vi "MCCETC03_Main.vi"() -> ()   [LabVIEW 2019]
uses:
  MCCETC_Global.vi
panel:
  out "T7":dbl format="%.2f"
  out "T6":dbl format="%.2f"
  out "T5":dbl format="%.2f"
  out "T4":dbl format="%.2f"
  in  "Logging":bool=TRUE
  out "status_rec":bool caption="Logging Status"
  out "T3":dbl format="%.2f"
  out "T2":dbl format="%.2f"
  in  "Tab Control":T1(tab)
  out "T0 Chart":waveform(dbl)[](graph)
  out "T1 Chart":waveform(dbl)[](graph)
  out "T2 Chart":waveform(dbl)[](graph)
  out "T3 Chart":waveform(dbl)[](graph)
  out "status_dio":bool caption="DIO Control Status"
  in  "degC_low":dbl=5.0 caption="From"
  in  "degC_hi":dbl=45.0 caption="To"
  out "alarm_t":bool caption="Temperature Alarm"
  out "T5 Chart":waveform(dbl)[](graph)
  out "T4 Chart":waveform(dbl)[](graph)
  out "T6 Chart":waveform(dbl)[](graph)
  out "T7 Chart":waveform(dbl)[](graph)
  in  "Readout Interval":i32=5 caption="sec"
  out "T1":dbl format="%.2f"
  out "T0":dbl format="%.2f"
  out "Readout Status":bool
  out "Last Measured":timestamp format="%<%Y-%m-%d %H:%M:%S>T"
  in  "stop":bool
  # "MCC E-TC #03:  Thermocouples for Annealing & Microwave Control Systems"
  # "Annealing System"
  # "K"
  # "K"
  # "Microwave System"
  # "°C"
  # "EIO Tube"
  # "EIO Top"
  # "°C"
  # "North He Riser:"
  # "°C"
  # "IVC Top:"
  # "°C"
  # "Heat Tape: IVC:"
  # "°F"
  # "Heat Tape: Turret:"
  # "°F"
  # "Good Temperature Range (degC)"
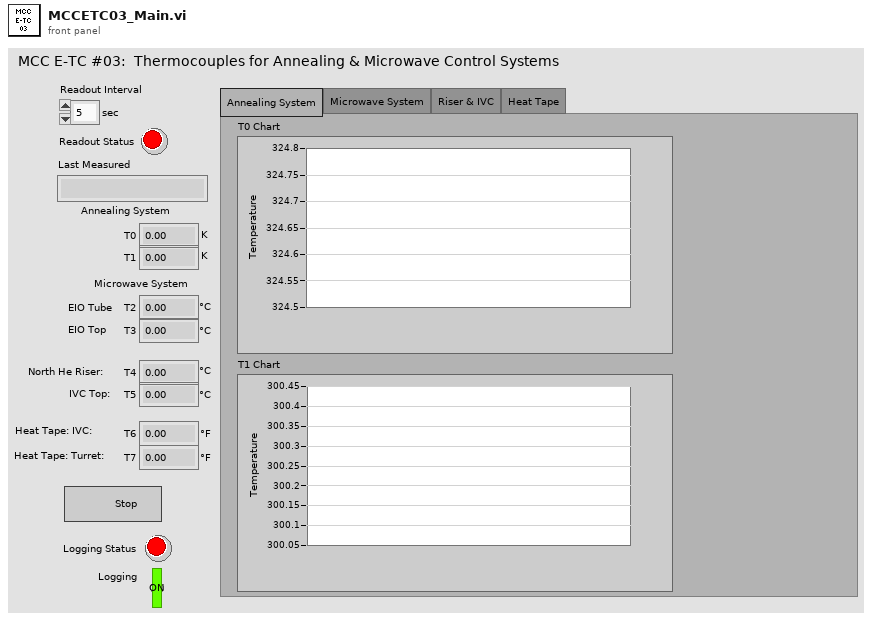
[diagram p1: front panel]
types:
  T1 = enum32{"Annealing System", "Microwave System", "Riser & IVC", "Heat Tape"}
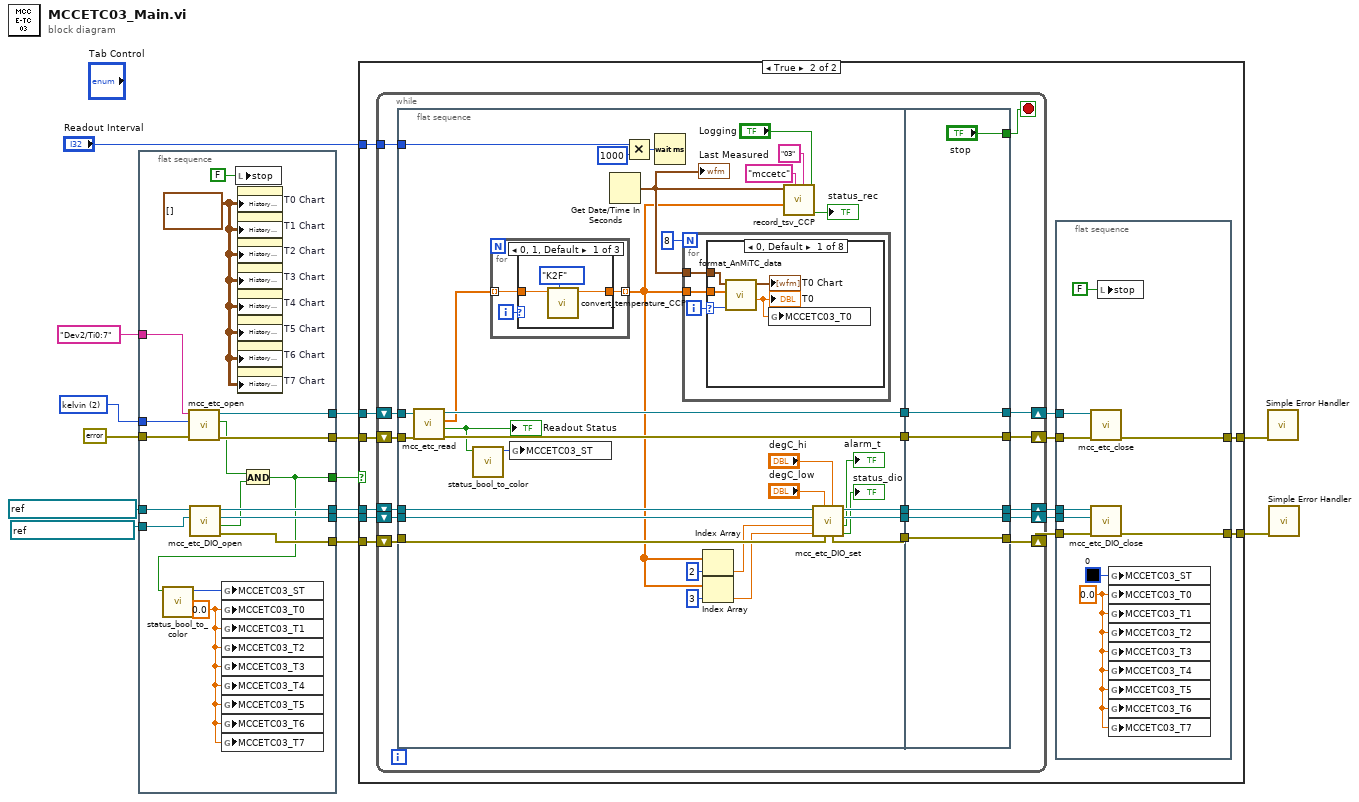
[diagram p0: block diagram]
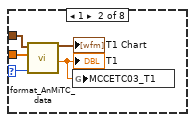
[diagram p3: hidden frame]
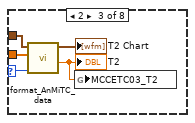
[diagram p4: hidden frame]
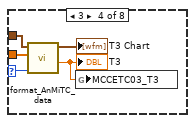
[diagram p5: hidden frame]
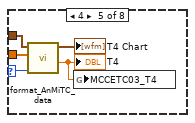
[diagram p6: hidden frame]
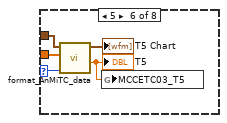
[diagram p7: hidden frame]
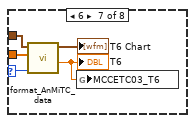
[diagram p8: hidden frame]
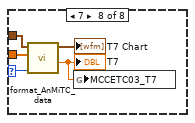
[diagram p9: hidden frame]
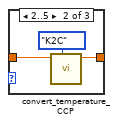
[diagram p10: hidden frame]
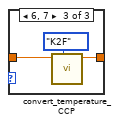
[diagram p11: hidden frame]
diagram:
  w10 = 2 items=["degC", "degF", "kelvin", "raw"] ("units")
  n1 = flat-sequence {
    tunnel: [w31] -> w14
    tunnel: errorcluster {"status"=FALSE, "code"=0, "source"=""} ("error in") -> [w30]
    tunnel: [w29] -> w12
    tunnel: "Dev2/Ti0:7" ("Device/Channel Name") -> [w28]
    tunnel: w10 -> [w27]
    tunnel: refnum<k21> "Dev2/AuxPort/Do0" ("output_line") -> [w26]
    tunnel: refnum<k21> "Dev2/AuxPort/Di4" ("input_line") -> [w25]
    tunnel: [w24] -> w6
    tunnel: [w23] -> w5
    tunnel: [w20] -> w2
    tunnel: [w15] -> w1
    frame #0 {
      w17 = 0.0 ("MCCETC01_T0")
      w18 = waveform(dbl)[][] [] ("History Data")
      n2 = call "mcc_etc_open.vi"("error in"=w30, "units"=w27, "name"=w28) -> ("error out"=w29:errorcluster, "status"=w22:bool, "task out"=w31:refnum<k24>)  [unwired: 6 in]
      n3 = call "mcc_etc_DIO_open.vi"("input_line"=w25, "output_line"=w26) -> ("error out"=w20:errorcluster, "status"=w21:bool, "input_task_out"=w23:refnum<k24>, "output_task out"=w24:refnum<k24>)  [unwired: 6 in]
      n4 = global write "MCCETC_Global.vi" "MCCETC03_T0"(w17) -> ()
      n5 = global write "MCCETC_Global.vi" "MCCETC03_T1"(w17) -> ()
      n6 = global write "MCCETC_Global.vi" "MCCETC03_T2"(w17) -> ()
      n7 = global write "MCCETC_Global.vi" "MCCETC03_T3"(w17) -> ()
      n8 = global write "MCCETC_Global.vi" "MCCETC03_T4"(w17) -> ()
      n9 = global write "MCCETC_Global.vi" "MCCETC03_T5"(w17) -> ()
      n10 = global write "MCCETC_Global.vi" "MCCETC03_T6"(w17) -> ()
      n11 = global write "MCCETC_Global.vi" "MCCETC03_T7"(w17) -> ()
      n12 = local write "stop"(FALSE ("Stop")) -> ()
      n13 = property on="T0 Chart" class="WFChart (strict)"("History Data"=w18) -> ()  [unwired: 2 in, 2 out]
      n14 = property on="T1 Chart" class="WFChart (strict)"("History Data"=w18) -> ()  [unwired: 2 in, 2 out]
      n15 = property on="T2 Chart" class="WFChart (strict)"("History Data"=w18) -> ()  [unwired: 2 in, 2 out]
      n16 = property on="T3 Chart" class="WFChart (strict)"("History Data"=w18) -> ()  [unwired: 2 in, 2 out]
      n17 = property on="T4 Chart" class="WFChart (strict)"("History Data"=w18) -> ()  [unwired: 2 in, 2 out]
      n18 = property on="T5 Chart" class="WFChart (strict)"("History Data"=w18) -> ()  [unwired: 2 in, 2 out]
      n19 = property on="T6 Chart" class="WFChart (strict)"("History Data"=w18) -> ()  [unwired: 2 in, 2 out]
      n20 = property on="T7 Chart" class="WFChart (strict)"("History Data"=w18) -> ()  [unwired: 2 in, 2 out]
      n21 = And(x=w22, y=w21) -> (x .and. y?=w15:bool)
      n22 = call "status_bool_to_color.vi"("status_bool_1"=w15) -> ("status_color"=w16:u32)  [unwired: 10 in]
      n23 = global write "MCCETC_Global.vi" "MCCETC03_ST"(w16) -> ()
    }
  }
  n24 = case shown="True" w1 {
    tunnel: w14 -> [_ w46]
    tunnel: w12 -> [w33 w45]
    tunnel: "Readout Interval" -> [_ w42]
    tunnel: w6 -> [_ w41]
    tunnel: w5 -> [_ w40]
    tunnel: [w32 w37] -> w4
    tunnel: [w33 w36] -> w3
    tunnel: w2 -> [w32 w35]
    frame False {
    }
    frame True {
      n25 = while {
        shift-right: [w71] -> w43
        shift-left: w45 -> [w72]
        shift-right: [w70] -> w44
        shift-left: w46 -> [w73]
        tunnel: w42 -> [w69]
        shift-right: [w66] -> w39
        shift-left: w41 -> [w68]
        shift-right: [w65] -> w38
        shift-left: w40 -> [w67]
        shift-right: [w63] -> w34
        shift-left: w35 -> [w64]
        stop <- w57 stop-if-true
        n26 = flat-sequence {
          tunnel: w73 -> [w104]
          tunnel: w72 -> [w103]
          tunnel: w69 -> [w100]
          tunnel: w68 -> [w99]
          tunnel: w67 -> [w98]
          tunnel: w64 -> [w95]
          tunnel: [w102] -> w62
          tunnel: [w101] -> w61
          tunnel: [w97] -> w60
          tunnel: [w96] -> w59
          tunnel: [w94] -> w58
          tunnel: [w161] -> w63
          tunnel: [w162] -> w65
          tunnel: [w163] -> w66
          tunnel: [w164] -> w70
          tunnel: [w165] -> w71
          tunnel: w62 -> [w165]
          tunnel: w61 -> [w164]
          tunnel: w60 -> [w163]
          tunnel: w59 -> [w162]
          tunnel: w58 -> [w161]
          tunnel: ["stop"] -> w57
          frame #0 {
            n27 = call "mcc_etc_read.vi"("error in"=w103, "task in"=w104) -> ("error out"=w102:errorcluster, "status"=w81:bool, "temperature_array"=w83:dbl[], "task out"=w101:refnum<k24>)  [unwired: 6 in]
            "Readout Status" <- w81
            n28 = call "status_bool_to_color.vi"("status_bool_1"=w81) -> ("status_color"=w82:u32)  [unwired: 10 in]
            n29 = for {
              tunnel: w83 -> [w150] mode=indexing
              tunnel: [w149] -> w75 mode=indexing
              i -> [w148]
              n30 = case shown="0, 1, Default" w148 {
                tunnel: w150 -> [w152 w156 w159]
                tunnel: [w151 w155 w158] -> w149
                frame 0, 1, Default {
                  n31 = call "convert_temperature_CCP.vi"("conv_type"=enum16{"None", "K2C", "K2F"}."K2F", "T_in"=w152) -> ("T_out"=w151:dbl)  [unwired: 9 in]
                }
                frame 2..5 {
                  n32 = call "convert_temperature_CCP.vi"("conv_type"=enum16{"None", "K2C", "K2F"}."K2C", "T_in"=w156) -> ("T_out"=w155:dbl)  [unwired: 9 in]
                }
                frame 6, 7 {
                  n33 = call "convert_temperature_CCP.vi"("conv_type"=enum16{"None", "K2C", "K2F"}."K2F", "T_in"=w159) -> ("T_out"=w158:dbl)  [unwired: 9 in]
                }
              }
            }
            n34 = global write "MCCETC_Global.vi" "MCCETC03_ST"(w82) -> ()
            n35 = Get Date/Time In Seconds() -> (seconds since 1Jan1904=w79:timestamp)
            "Last Measured" <- w79
            n36 = Multiply(x=w100, y=1000) -> (x*y=w89:i32)
            n37 = Wait (ms)(milliseconds to wait=w89) -> ()  [unwired: 1 out]
            n38 = for {
              N: 8 -> [_]
              tunnel: w75 -> [w106]
              tunnel: w79 -> [w105]
              i -> [w107]
              n39 = case shown="0, Default" w107 {
                selector: w107 -> [w111 w116 w121 w126 w131 w136 w141 w146]
                tunnel: w106 -> [w112 w117 w122 w127 w132 w137 w142 w147]
                tunnel: w105 -> [w110 w115 w120 w125 w130 w135 w140 w145]
                frame 0, Default {
                  n40 = call "format_AnMiTC_data.vi"("index"=w111, "value_array"=w112, "time"=w110) -> ("value"=w108:dbl, "waveform_array"=→"T0 Chart":waveform(dbl)[])  [unwired: 7 in]
                  "T0" <- w108
                  n41 = global write "MCCETC_Global.vi" "MCCETC03_T0"(w108) -> ()
                }
                frame 1 {
                  n42 = call "format_AnMiTC_data.vi"("index"=w116, "value_array"=w117, "time"=w115) -> ("value"=w113:dbl, "waveform_array"=→"T1 Chart":waveform(dbl)[])  [unwired: 7 in]
                  "T1" <- w113
                  n43 = global write "MCCETC_Global.vi" "MCCETC03_T1"(w113) -> ()
                }
                frame 2 {
                  n44 = call "format_AnMiTC_data.vi"("index"=w121, "value_array"=w122, "time"=w120) -> ("value"=w118:dbl, "waveform_array"=→"T2 Chart":waveform(dbl)[])  [unwired: 7 in]
                  "T2" <- w118
                  n45 = global write "MCCETC_Global.vi" "MCCETC03_T2"(w118) -> ()
                }
                frame 3 {
                  n46 = call "format_AnMiTC_data.vi"("index"=w126, "value_array"=w127, "time"=w125) -> ("value"=w123:dbl, "waveform_array"=→"T3 Chart":waveform(dbl)[])  [unwired: 7 in]
                  "T3" <- w123
                  n47 = global write "MCCETC_Global.vi" "MCCETC03_T3"(w123) -> ()
                }
                frame 4 {
                  n48 = call "format_AnMiTC_data.vi"("index"=w131, "value_array"=w132, "time"=w130) -> ("value"=w128:dbl, "waveform_array"=→"T4 Chart":waveform(dbl)[])  [unwired: 7 in]
                  "T4" <- w128
                  n49 = global write "MCCETC_Global.vi" "MCCETC03_T4"(w128) -> ()
                }
                frame 5 {
                  n50 = call "format_AnMiTC_data.vi"("index"=w136, "value_array"=w137, "time"=w135) -> ("value"=w133:dbl, "waveform_array"=→"T5 Chart":waveform(dbl)[])  [unwired: 7 in]
                  "T5" <- w133
                  n51 = global write "MCCETC_Global.vi" "MCCETC03_T5"(w133) -> ()
                }
                frame 6 {
                  n52 = call "format_AnMiTC_data.vi"("index"=w141, "value_array"=w142, "time"=w140) -> ("value"=w138:dbl, "waveform_array"=→"T6 Chart":waveform(dbl)[])  [unwired: 7 in]
                  "T6" <- w138
                  n53 = global write "MCCETC_Global.vi" "MCCETC03_T6"(w138) -> ()
                }
                frame 7 {
                  n54 = call "format_AnMiTC_data.vi"("index"=w146, "value_array"=w147, "time"=w145) -> ("value"=w143:dbl, "waveform_array"=→"T7 Chart":waveform(dbl)[])  [unwired: 7 in]
                  "T7" <- w143
                  n55 = global write "MCCETC_Global.vi" "MCCETC03_T7"(w143) -> ()
                }
              }
            }
            n56 = Index Array(array=w75, index=2) -> (element=w77:dbl)
            n57 = Index Array(array=w75, index=3) -> (element=w74:dbl)
            n58 = call "record_tsv_CCP.vi"("logging_on"="Logging", "file_name"="03", "folder_name"="mccetc", "value_array"=w75, "time"=w79) -> ("status_log"=→"status_rec":bool)  [unwired: 5 in, 1 out]
            n59 = call "mcc_etc_DIO_set.vi"("degC_hi"="degC_hi", "error in"=w95, "degC_low"="degC_low", "degC_ch2"=w74, "degC_ch1"=w77, "input_line"=w98, "output_line"=w99) -> ("DIO_control_status"=→"status_dio":bool, "alarm"=→"alarm_t":bool, "input_line_out"=w96:refnum<k24>, "output_line_out"=w97:refnum<k24>, "error out"=w94:errorcluster)
          }
          frame #1 {
          }
        }
      }
      n60 = flat-sequence {
        tunnel: w44 -> [w56]
        tunnel: w43 -> [w55]
        tunnel: w39 -> [w54]
        tunnel: w38 -> [w53]
        tunnel: [w52] -> w37
        tunnel: [w51] -> w36
        tunnel: w34 -> [w50]
        frame #0 {
          w48 = 0.0 ("MCCETC01_T0")
          n61 = call "mcc_etc_close.vi"("error in"=w55, "task in"=w56) -> ("error out"=w51:errorcluster)  [unwired: 8 in, 1 out]
          n62 = call "mcc_etc_DIO_close.vi"("error in"=w50, "input_line"=w53, "output_line"=w54) -> ("error out"=w52:errorcluster)  [unwired: 8 in]
          n63 = local write "stop"(FALSE ("Stop")) -> ()
          n64 = global write "MCCETC_Global.vi" "MCCETC03_ST"(u32 0 ("MCCETC03_ST")) -> ()
          n65 = global write "MCCETC_Global.vi" "MCCETC03_T0"(w48) -> ()
          n66 = global write "MCCETC_Global.vi" "MCCETC03_T1"(w48) -> ()
          n67 = global write "MCCETC_Global.vi" "MCCETC03_T2"(w48) -> ()
          n68 = global write "MCCETC_Global.vi" "MCCETC03_T3"(w48) -> ()
          n69 = global write "MCCETC_Global.vi" "MCCETC03_T4"(w48) -> ()
          n70 = global write "MCCETC_Global.vi" "MCCETC03_T5"(w48) -> ()
          n71 = global write "MCCETC_Global.vi" "MCCETC03_T6"(w48) -> ()
          n72 = global write "MCCETC_Global.vi" "MCCETC03_T7"(w48) -> ()
        }
      }
    }
  }
  n73 = call <vilib>:"Simple Error Handler.vi"("error in (no error)"=w3) -> ()  [unwired: 4 in, 5 out]
  n74 = call <vilib>:"Simple Error Handler.vi"("error in (no error)"=w4) -> ()  [unwired: 4 in, 5 out]
